vi "QTrkSetZLUTBiasTable.vi"(8 "error in (no error)":errorcluster, 11 "QTrk Instance":T1) -> (0 "error out":errorcluster, 1 "Bias correction table":sgl[][](array[numeric]), 3 "QTrk Instance":T1)   [LabVIEW 2011]
uses:
  QTrkInstance.ctl
  QTrkDLL.vi
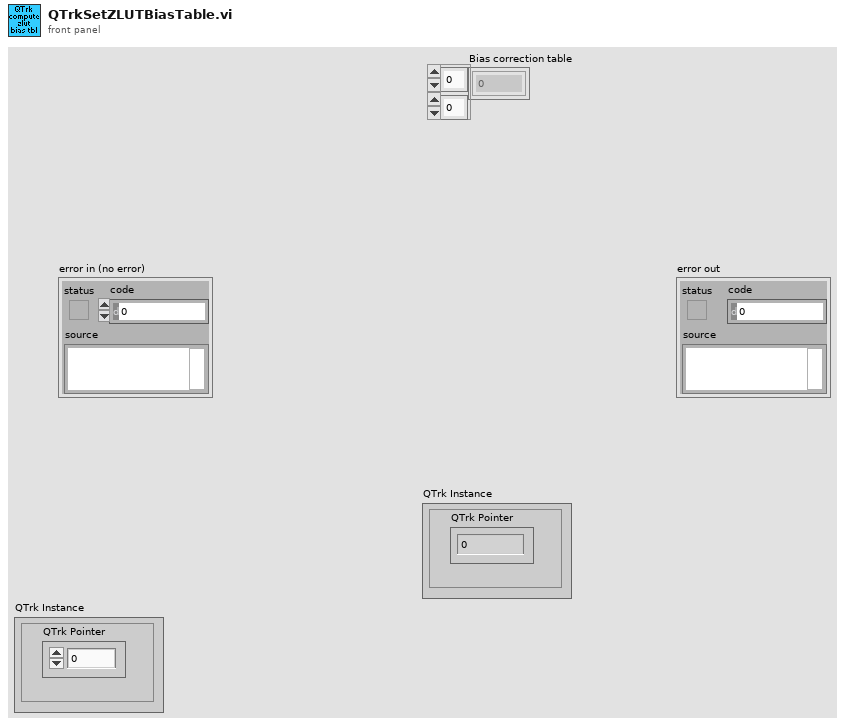
[diagram p1: front panel]
types:
  T1 = typedef "QTrkInstance.ctl" = cluster{"QTrk Pointer":u64}
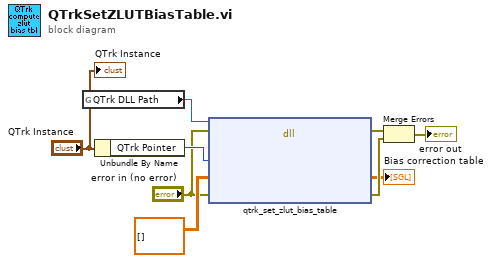
[diagram p0: block diagram]
diagram:
  n1 = global read "QTrkDLL.vi" "QTrk DLL Path"() -> (w7:path)
  n2 = Unbundle By Name("QTrk Instance") -> ("QTrk Pointer"=w8:u64)
  n3 = dll-call lib="D:/jcnossen1/cudaqi-tracker/bin/jtrk-labview.dll" fn="qtrk_set_zlut_bias_table"(path in=w7, error in="error in (no error)", "tracker"=w8, "table"=sgl[][] [] ("Bias correction table"), "error"="error in (no error)") -> (error out=w5:errorcluster, "table"=→"Bias correction table":sgl[][], "error"=w6:errorcluster)  [unwired: 3 in, 1 out]
  n4 = Merge Errors(w5, w6) -> (→"error out":errorcluster)
  "QTrk Instance" <- "QTrk Instance"
